vi "Main.vi"() -> ()   [LabVIEW 2021]
uses:
  Strict Type Controls/Command.ctl
  classes/Tushars Events Toolkit/Software/Modules/EventClient_ObjectReference.ctl
  Strict Type Controls/Settings Operation.ctl
  Strict Type Controls/Settings.ctl
  1f5d9b14-0bda-4edd-bf62-f35b82af222a.vi
  classes/Variable Manager/VariableManager_Bool.vi
  <vilib>/Utility/file.llb/Write To Spreadsheet File (string).vi
  classes/Variable Manager/VariableManager_Double.vi
  classes/Variable Manager/VariableManager_String.vi
panel:
  out "filterSetup?":bool
  out "Quit":bool
  out "error out":errorcluster
  in  "error in (no error)":errorcluster
  in  "abort":bool
  in  "start":bool
  out "gratSetup?":bool
  out "Status":string
  in  "Port Set":bool
  in  "Merlin":refnum<visa-resource-name>
  in  "Mono":refnum<visa-resource-name>
  out "statusFilter":bool
  in  "Start Filter Wheel":bool
  out "Agilent Current":dbl format="%#.4f A"
  out "Agilent Voltage":dbl format="%#.4f V"
  out "Test Status":bool
  out "statusMerlin":bool
  out "statusMC":bool
  out "statusPS":bool
  out "statusSM":bool
  in  "Start Merlin":bool
  in  "Start Monochromator":bool
  in  "Start Power Supply":bool
  in  "Start Source Meter":bool
  out "Merlin Voltage":dbl format="%#.7f mV"
  out "Measuring Wavelength":dbl format="%#.7f nm"
  out "Source Meter Voltage":dbl format="%#.7f mV"
  in  "tab":T1(tab)=enum."Script"
  in  "exportVT":bool
  out "VTGraph":cluster{dbl[], dbl[]}(graph)
  in  "Test Mode":enum16{"Time Mode", "dV/dt Mode"}(ring)
  in  "Log Interval":u32=50 min=100 step=1 format="%.0f mSec"
  in  "Test Time":dbl step=1.0 format="%<%H:%M:%S>t"
  out "Time Remaining":dbl format="%<%H:%M:%S>t"
  in  "Target dV/dt":dbl format="%#.9f mV"
  in  "Lock In time":dbl step=1.0 format="%<%H:%M:%S>t"
  out "dV/dt":dbl format="%#.11f mV"
  out "Locked Time":dbl step=1.0 format="%<%H:%M:%S>t"
  in  "Perform Test After":T1(ring)=enum."Voltage Vs Wavelength"
  out "Wave":bool
  out "Slit":bool
  out "Shutter":bool
  out "Filter":bool
  out "Gr.Den":bool
  in  "GratingNo":i32=1 min=1 max=3 step=1
  in  "Wavelen(nm)":i32
  in  "setWavelength":bool
  in  "SetGrating":bool
  in  "SetSlit":bool
  in  "Slit":i32=1 min=1 max=8 step=1
  out "Wavenumber":i32
  in  "Set Grating Density":bool
  in  "GratingDen":i32=1 min=1 max=2 step=1
  in  "Filter Set":bool
  in  "Filter Num":i32=1 min=1 max=5 step=1
  in  "Shutter":enum16{"Open", "Close"}(ring)
  in  "ShutterOp":bool
  in  "Filter Block":bool
  in  "Filter Disable":bool
  in  "Filter Enab":bool
  in  "Frequency":u32=15 min=8 max=1100 step=1
  in  "setMerlin":bool
  in  "#Filter Stages":enum16{"None", "1 Pole", "2 Pole"}(ring)
  in  "Phase":enum16{"1 Phase", "2 Phase"}(ring)
  in  "SyncMode":T2(ring)
  in  "Time Const":T3(ring)
  in  "setOffsets":bool
  in  "portD":bool
  in  "portA":bool
  in  "Settling Time (ms)":dbl=10000.0
  in  "To":i32=1000
  in  "Step":dbl=100.0
  in  "From":i32=200
  in  "exportSweep":bool
  out "sweep":cluster{dbl[], dbl[]}[](graph)
  in  "Slit":string(combo)
  in  "Sweep Results":i32(listbox)
  in  "Reset":bool
  out "Gr.no":bool
  out "Reset 2":bool
  in  "exportScriptWave":bool
  out "scriptSweep":cluster{dbl[], dbl[]}[](graph)
  in  "Command":T4
  in  "Parm 4":dbl format="%#.6f"
  in  "Parm 3":dbl format="%#.6f"
  in  "openScript":bool
  in  "exportScript":bool
  in  "update":bool
  out "scriptGraph":cluster{dbl[], dbl[]}(graph)
  in  "Parm 2":dbl format="%#.6f"
  in  "Parm 1":dbl format="%#.6f"
  in  "script":i32(listbox)
  in  "add":bool
  in  "remove":bool
  in  "exportScriptResults":bool
  in  "Script Avg Interval":u32=200 min=100 step=1 format="%.0f mSec"
  # "Status"
  # "Port Setting"
  # "NOTE:\n1. if this LED is OFF then GPIB is not connected...\n2. Close program before power off Instruments..."
  # "Test Type"
  # "Test Time"
  # "Voltage Results"
  # "Monochromator"
  # "Merlin"
  # "Merlin"
  # "Sweep"
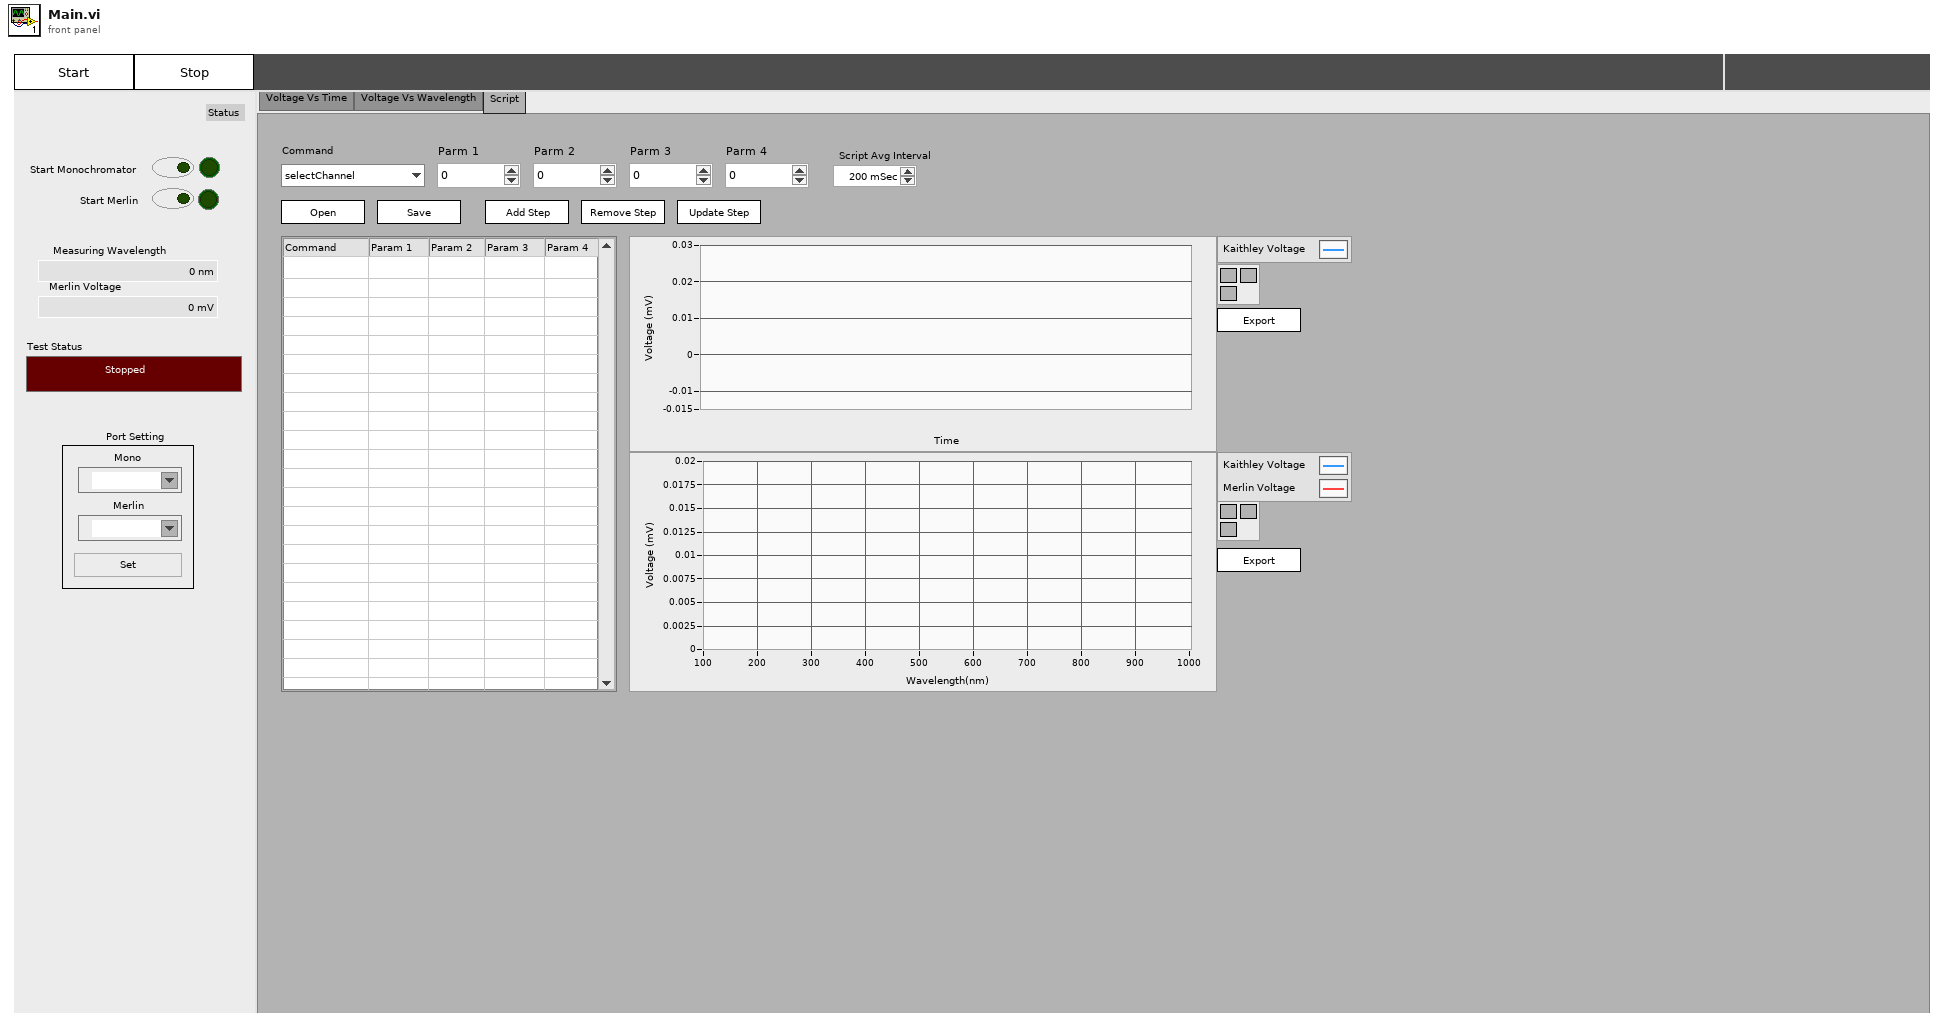
[diagram p1: front panel]
types:
  T1 = enum32{"Voltage Vs Time", "Voltage Vs Wavelength", "Script"}
  T2 = enum16{"Int Chop Off", "Int Chop On", "Ext Chop Off", "Ext Chop On"}
  T3 = enum16{".003s", ".010s", ".030s", ".100s", ".300s", "1.00s", "3.00s", "10.0s", "30.0s", "100s"}
  T4 = typedef "Command.ctl" = enum16{"selectChannel", "setDCVoltage", "setDCCurrent", "setVoltageSteps", "wait", "setWavelength", "setWavelengthSteps"}
  T5 = typedef "Settings Operation.ctl" = enum8{"Get Value", "Set Value", "Read File", "Write File", "Write Stored Value"}
  T6 = enum32{"invalid app kind", "Development System", "Run Time System", "Student Edition", "Embedded LabVIEW", "Evaluation", "Custom"}
  T7 = cluster{"startTime":u32, "lastUpdate":u32, "lastVoltage":dbl, "run?":bool, "From":i32, "time":dbl[], "MerlinVal":dbl[], "SMVolt":dbl[], "sweepType":enum16{"ASC", "DESC"}, "Wavlnth":dbl[], "Test Mode":enum16{"Time Mode", "dV/dt Mode"}, "tab":enum32{"Voltage Vs Time", "Voltage Vs Wavelength", "Script"}, "script":string[][], "dV/dt":dbl[], "graphUpdate":u32, "Filter Num":i32}
  T8 = typedef "EventClient_ObjectReference.ctl" = refnum<k1>
  T9 = typedef "Settings.ctl" = cluster{"Mono Cr":cluster{"Port":refnum<visa-resource-name>, "baud rate":u32, "data bits":u16, "parity":enum16{"None", "Odd", "Even", "Mark", "Space"}, "stop bits":u16, "flow control":u16, "timeout":u32}, "Merlin":cluster{"Port":refnum<visa-resource-name>, "baud rate":u32, "data bits":u16, "parity":enum16{"None", "Odd", "Even", "Mark", "Space"}, "stop bits":u16, "flow control":u16, "timeout":u32}}
  T10 = cluster{"#Stages":enum16{"None", "1 Pole", "2 Pole"}, "Phase":enum16{"1 Phase", "2 Phase"}, "SyncMode":enum16{"Int Chop Off", "Int Chop On", "Ext Chop Off", "Ext Chop On"}, "Time Const":enum16{".003s", ".010s", ".030s", ".100s", ".300s", "1.00s", "3.00s", "10.0s", "30.0s", "100s"}, "Frequency":u32}
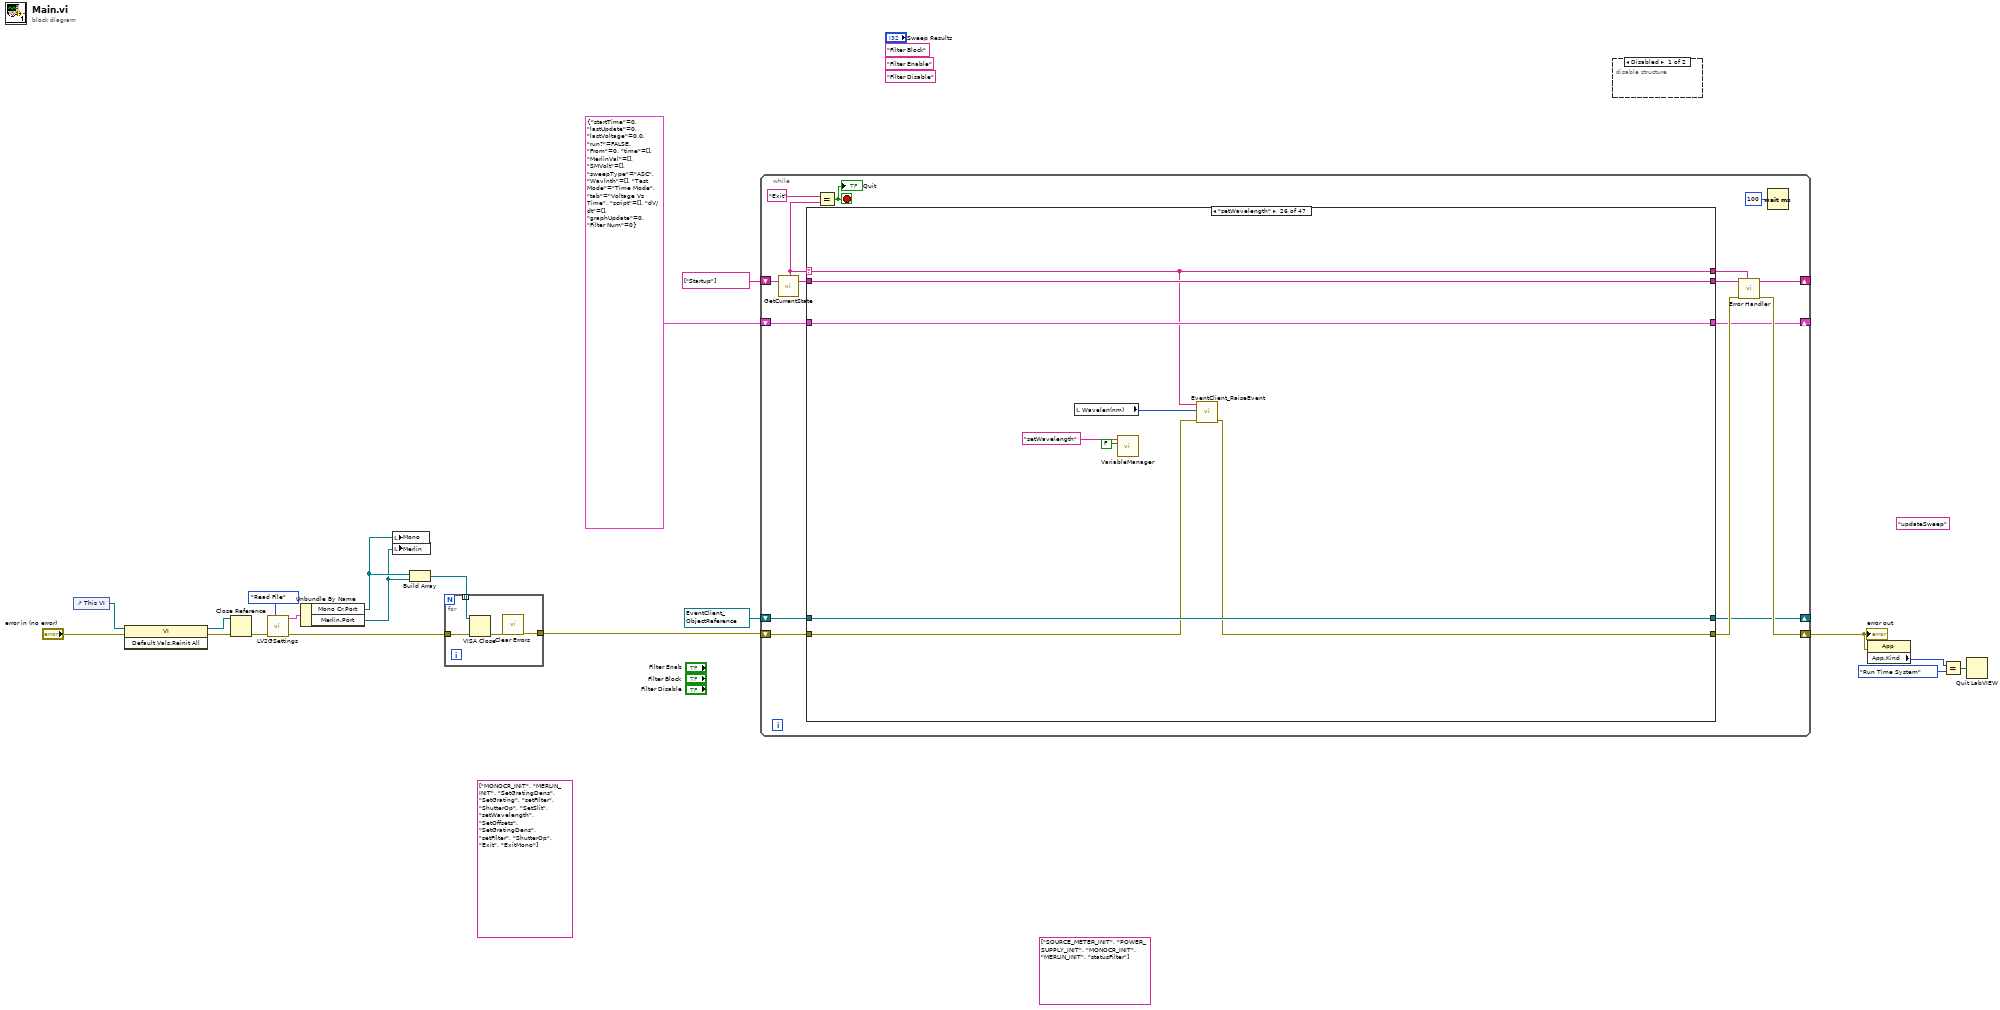
[diagram p0: block diagram]
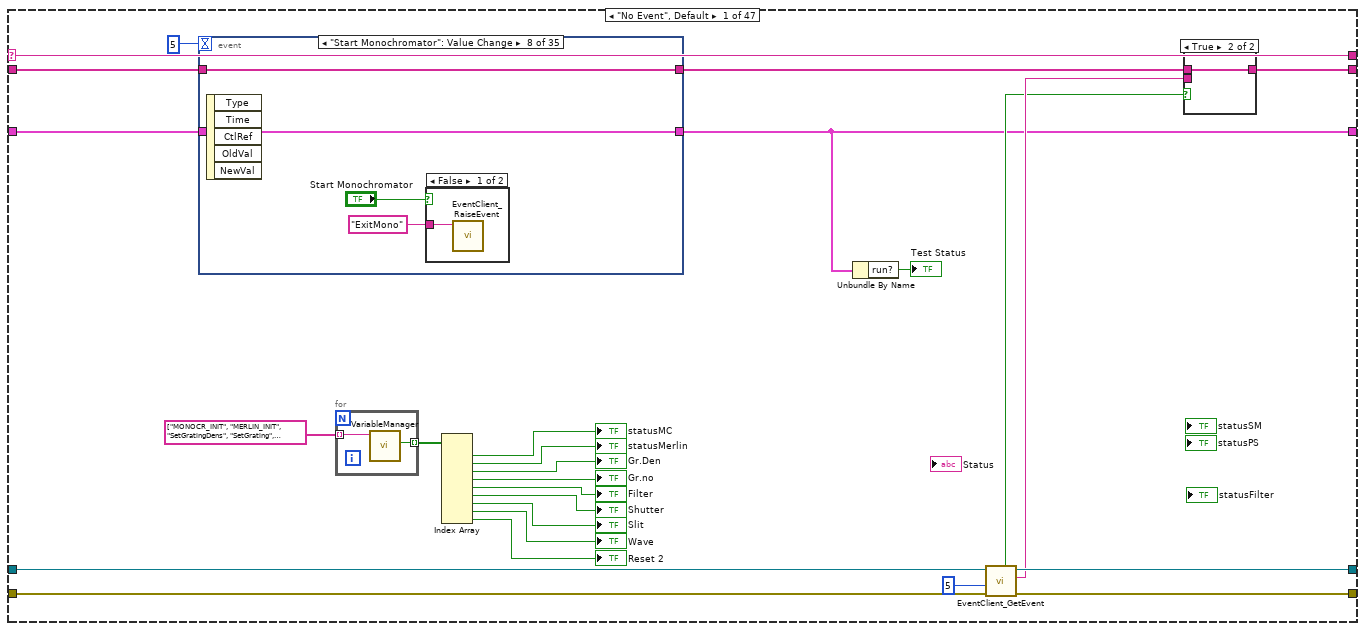
[diagram p3: hidden frame]
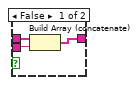
[diagram p4: hidden frame]
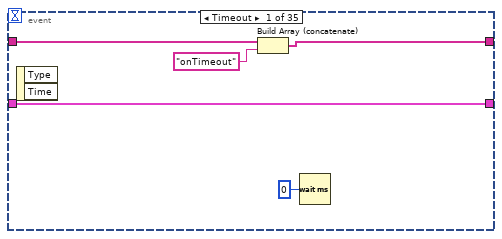
[diagram p5: hidden frame]
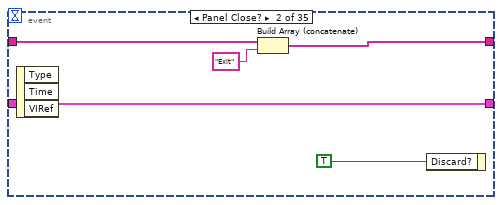
[diagram p6: hidden frame]
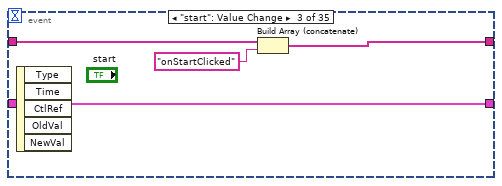
[diagram p7: hidden frame]
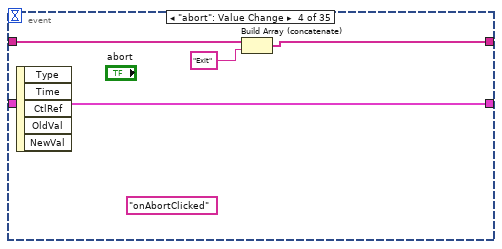
[diagram p8: hidden frame]
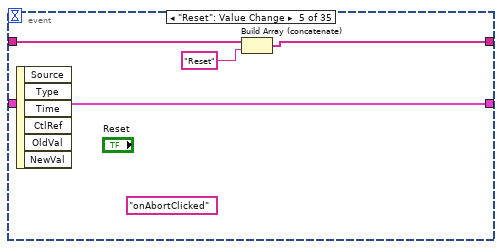
[diagram p9: hidden frame]
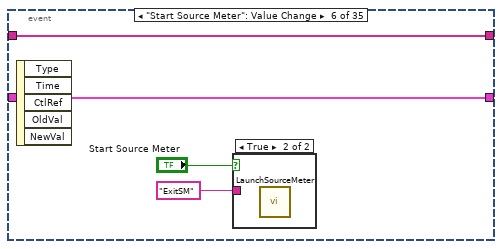
[diagram p10: hidden frame]
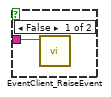
[diagram p11: hidden frame]
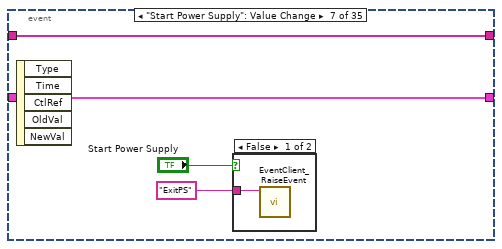
[diagram p12: hidden frame]
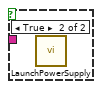
[diagram p13: hidden frame]
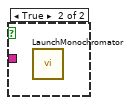
[diagram p14: hidden frame]
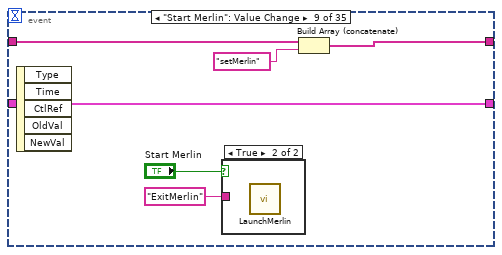
[diagram p15: hidden frame]
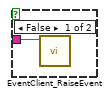
[diagram p16: hidden frame]
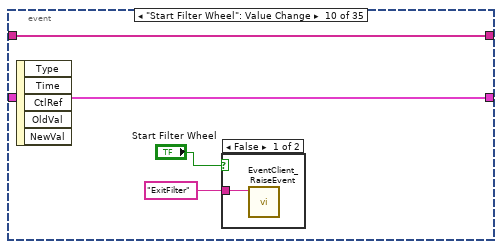
[diagram p17: hidden frame]
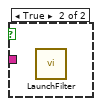
[diagram p18: hidden frame]
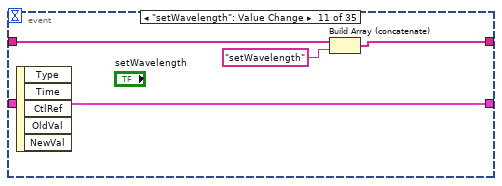
[diagram p19: hidden frame]
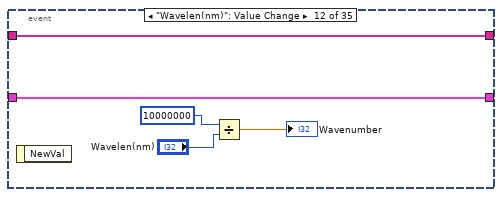
[diagram p20: hidden frame]
diagram:
  (unwired) "updateSweep" ("String")
  (unwired) string[] ["MONOCR_INIT", "MERLIN_INIT", "SetGratingDens", "SetGrating", "setFIlter", "ShutterOp", "SetSlit", "setWavelength", "SetOffsets", "SetGratingDens", "setFIlter", "ShutterOp", "Exit", "ExitMono"] ("Events")
  (unwired) string[] ["SOURCE_METER_INIT", "POWER_SUPPLY_INIT", "MONOCR_INIT", "MERLIN_INIT", "statusFilter"] ("State Array Out")
  (unwired) "Filter Block"
  (unwired) "Filter Disable"
  (unwired) "Filter Enable"
  w19 = T8 refnum items=["EventClient"] ("reference")
  n1 = control-ref of="This VI"() -> (w11:refnum<vi>)
  n2 = invoke class="VI" method="Default Vals.Reinit All"(reference=w11, error in="error in (no error)") -> (reference out=w9:refnum<vi>, error out=w10:errorcluster)  [unwired: 1 in, 1 out]
  n3 = Close Reference(reference=w9, error in (no error)=w10) -> (error out=w8:errorcluster)
  n4 = call "LV2GSettings.vi"("Operation"=Settings_Operation."Read File", "error in (no error)"=w8) -> ("error out"=w3:errorcluster, "Settings out"=w7:T9)  [unwired: 8 in]
  n5 = Unbundle By Name(w7) -> ("Mono Cr.Port"=w5:refnum<visa-resource-name>, "Merlin.Port"=w4:refnum<visa-resource-name>)
  n6 = local write "Mono"(w5) -> ()
  n7 = local write "Merlin"(w4) -> ()
  n8 = Build Array(w5, w4) -> (w2:refnum<visa-resource-name>[])
  n9 = for {
    tunnel: w3 -> [w22]
    tunnel: w2 -> [w23] mode=indexing
    tunnel: [w20] -> w1
    n10 = VISA Close(VISA resource name=w23, error in (no error)=w22) -> (error out=w21:errorcluster)
    n11 = call <vilib>:"Clear Errors.vi"("error in (no error)"=w21) -> ("error out"=w20:errorcluster)  [unwired: 5 in, 1 out]
  }
  n12 = while {
    shift-right: [w35] -> _
    shift-left: string[] ["Startup"] ("State Array Out") -> [w39]
    shift-right: [w31] -> w16
    shift-left: w1 -> [w32]
    shift-right: [w28] -> _
    shift-left: w19 -> [w27]
    shift-right: [w25] -> _
    shift-left: T7 {"startTime"=0, "lastUpdate"=0, "lastVoltage"=0.0, "run?"=FALSE, "From"=0, "time"=[], "MerlinVal"=[], "SMVolt"=[], "sweepType"=enum."ASC", "Wavlnth"=[], "Test Mode"=enum."Time Mode", "tab"=enum."Voltage Vs Time", "script"=[], "dV/dt"=[], "graphUpdate"=0, "Filter Num"=0} -> [w26]
    stop <- w36 stop-if-true
    n13 = call "GetCurrentState.vi"("State Array In"=w39) -> ("Current State"=w29:string, "State Array Out"=w38:string[])  [unwired: 17 in]
    n14 = case shown="\"setWavelength\"" w29 {
      selector: w29 -> [w65 w246 w258 w268 w273 w278 w283 w288 w306 w322 w345 w372 w390 w401 w422 w439 w447 w477 w495 w506 w518 w526 w532 w541 w552 w561 w571 w579 w588 w604 w617 w623 w633 w662 w673 w678 w699 w754 w774 w804 w836 w864 w922 w984 w1019 w1048 w1064]
      tunnel: w38 -> [w64 w245 w264 w269 w274 w279 w284 w289 w307 w323 w346 w373 w391 w402 w423 w440 w448 w450 w496 w507 w519 w527 w536 w545 w556 w565 w574 w583 w592 w608 w619 w624 w634 w663 w674 w679 w690 w737 w758 w796 w828 w855 w901 w985 w1020 w1047 w1051]
      tunnel: [w55 w244 w264 w269 w274 w279 w284 w289 w307 w323 w346 w373 w391 w402 w423 w440 w448 w449 w496 w507 w519 w527 w536 w545 w556 w565 w574 w583 w592 w608 w619 w624 w634 w663 w674 w679 w691 w736 w757 w795 w830 w854 w900 w973 w1020 w1047 w1051] -> w34
      tunnel: [w60 w238 w259 w267 w272 w277 w282 w287 w305 w321 w344 w371 w389 w400 w421 w438 w446 w476 w494 w505 w512 w520 w533 w542 w553 w559 w568 w577 w587 w605 w614 w622 w629 w658 w669 w677 w698 w753 w773 w803 w835 w862 w902 w980 w1018 w1046 errorcluster {"status"=FALSE, "code"=0, "source"=""} ("error in (no error)")] -> w30
      tunnel: [w65 w246 w258 w268 w273 w278 w283 w288 w306 w322 w345 w372 w390 w401 w422 w439 w447 w477 w495 w506 w518 w526 w532 w541 w552 w561 w571 w579 w588 w604 w617 w623 w633 w662 w673 w678 w699 w754 w774 w804 w836 w864 w922 w984 w1019 w1048 w1064] -> w33
      tunnel: w32 -> [w61 w226 w262 w267 w272 w277 w282 w287 w305 w321 w344 w371 w389 w400 w421 w438 w446 w476 w494 w505 w513 w521 w534 w543 w554 w560 w570 w580 w589 w606 w615 w622 w631 w660 w671 w677 w698 w753 w773 w803 w835 w862 w903 w981 w1018 w1046 w1052]
      tunnel: [w59 w236 w261 w266 w271 w276 w281 w286 w304 w320 w343 w370 w388 w399 w420 w437 w445 w475 w493 w504 w517 w525 w535 w544 w555 w564 w573 w582 w591 w607 w618 w621 w627 w656 w667 w676 w697 w752 w772 w802 w834 w863 w921 w983 w1017 w1045 w1050] -> w28
      tunnel: w27 -> [w62 _ w263 w266 w271 w276 w281 w286 w304 w320 w343 w370 w388 w399 w420 w437 w445 w475 w493 w504 w517 w525 w535 w544 w555 w564 w573 w582 w591 w607 w618 w621 w632 w661 w672 w676 w697 w752 w772 w802 w834 w863 w921 w983 w1017 w1045 w1050]
      tunnel: w26 -> [w53 w234 w257 w265 w270 w275 w280 w285 w303 w319 w342 w369 w387 w398 w419 w436 w444 w474 w492 w503 w516 w524 w530 w540 w551 w563 w572 w581 w590 w597 w616 w620 w625 w655 w666 w675 w696 w742 w771 w800 w833 w857 w920 w971 w1010 w1044 w1049]
      tunnel: [w52 w234 w257 w265 w270 w275 w280 w285 w303 w319 w342 w369 w387 w398 w419 w436 w444 w473 w491 w503 w516 w524 w530 w540 w551 w563 w572 w581 w590 w597 w616 w620 w625 w655 w666 w675 w696 w741 w768 w798 w833 w856 w919 w982 w1009 w1044 w1049] -> w25
      frame "No Event", Default {
        n15 = event shown="[7] \"Start Monochromator\": Value Change" {
          selector: _ -> [_ _ _ _ _ _ _ _ _ _ _ _ _ _ _ _ _ _ _ _ _ _ _ _ _ _ _ _ _ _ _ _ _ _ _]
          dyn-events: _ -> [_ _ _ _ _ _ _ _ _ _ _ _ _ _ _ _ _ _ _ _ _ _ _ _ _ _ _ _ _ _ _ _ _ _ _]
          timeout: 5 -> [_ _ _ _ _ _ _ _ _ _ _ _ _ _ _ _ _ _ _ _ _ _ _ _ _ _ _ _ _ _ _ _ _ _ _]
          tunnel: [w74 w79 w84 w88 w92 w97 w102 w107 w110 w119 w123 w129 w132 w136 w140 w144 w147 w151 w155 w159 w163 w167 w171 w175 w179 w183 w187 w191 w195 w199 w203 w207 w211 w215 w219] -> w56
          tunnel: w64 -> [w76 w81 w85 w89 w93 w97 w102 w107 w114 w119 w124 w129 w133 w137 w141 w145 w148 w152 w156 w159 w164 w168 w172 w176 w180 w184 w188 w192 w196 w200 w204 w208 w212 w216 w220]
          tunnel: w53 -> [w75 w77 w82 w87 w91 w96 w101 w106 w113 w118 w121 w128 w130 w134 w138 w142 w149 w153 w157 w160 w161 w165 w169 w173 w177 w181 w185 w189 w193 w197 w201 w205 w209 w213 w217]
          tunnel: [w75 w77 w82 w87 w91 w96 w101 w106 w113 w118 w121 w128 w130 w134 w138 w142 w149 w153 w157 w160 w161 w165 w169 w173 w177 w181 w185 w189 w193 w197 w201 w205 w209 w213 w217] -> w52
          event Timeout {
            n16 = event-data() -> ()  [unwired: 1 in, 2 out]
            n17 = Build Array (concatenate)(w76, "onTimeout" ("x")) -> (w74:string[])
            n18 = Wait (ms)(milliseconds to wait=u32 0) -> ()  [unwired: 1 out]
          }
          event Panel Close? {
            n19 = event-data() -> ()  [unwired: 1 in, 3 out]
            n20 = Build Array (concatenate)(w81, "Exit" ("x")) -> (w79:string[])
            n21 = event-data("Discard?"=TRUE) -> ()  [unwired: 1 in, 1 out]
          }
          event "start": Value Change {
            n22 = event-data() -> ()  [unwired: 1 in, 5 out]
            n23 = Build Array (concatenate)(w85, "onStartClicked" ("x")) -> (w84:string[])
          }
          event "abort": Value Change {
            (unwired) "onAbortClicked" ("x")
            n24 = event-data() -> ()  [unwired: 1 in, 5 out]
            n25 = Build Array (concatenate)(w89, "Exit" ("x")) -> (w88:string[])
          }
          event "Reset": Value Change {
            (unwired) "onAbortClicked" ("x")
            n26 = event-data() -> ()  [unwired: 1 in, 6 out]
            n27 = Build Array (concatenate)(w93, "Reset" ("x")) -> (w92:string[])
          }
          event "Start Source Meter": Value Change {
            n28 = event-data() -> ()  [unwired: 1 in, 5 out]
            n29 = case shown="True" "Start Source Meter" {
              tunnel: "ExitSM" -> [w98 _]
              frame False {
                n30 = call "EventClient_RaiseEvent.vi"("Event"=w98) -> ()  [unwired: 10 in, 1 out]
              }
              frame True {
                n31 = call "LaunchSourceMeter.vi"() -> ()  [unwired: 11 in, 1 out]
              }
            }
          }
          event "Start Power Supply": Value Change {
            n32 = event-data() -> ()  [unwired: 1 in, 5 out]
            n33 = case shown="False" "Start Power Supply" {
              tunnel: "ExitPS" -> [w103 _]
              frame False {
                n34 = call "EventClient_RaiseEvent.vi"("Event"=w103) -> ()  [unwired: 10 in, 1 out]
              }
              frame True {
                n35 = call "LaunchPowerSupply.vi"() -> ()  [unwired: 11 in, 1 out]
              }
            }
          }
          event "Start Monochromator": Value Change {
            n36 = event-data() -> ()  [unwired: 1 in, 5 out]
            n37 = case shown="False" "Start Monochromator" {
              tunnel: "ExitMono" -> [w108 _]
              frame False {
                n38 = call "EventClient_RaiseEvent.vi"("Event"=w108) -> ()  [unwired: 10 in, 1 out]
              }
              frame True {
                n39 = call "LaunchMonochromator.vi"() -> ()  [unwired: 11 in, 1 out]
              }
            }
          }
          event "Start Merlin": Value Change {
            n40 = event-data() -> ()  [unwired: 1 in, 5 out]
            n41 = case shown="True" "Start Merlin" {
              tunnel: "ExitMerlin" -> [w115 _]
              frame False {
                n42 = call "EventClient_RaiseEvent.vi"("Event"=w115) -> ()  [unwired: 10 in, 1 out]
              }
              frame True {
                n43 = call "LaunchMerlin.vi"() -> ()  [unwired: 11 in, 1 out]
              }
            }
            n44 = Build Array (concatenate)(w114, "setMerlin") -> (w110:string[])
          }
          event "Start Filter Wheel": Value Change {
            n45 = event-data() -> ()  [unwired: 1 in, 5 out]
            n46 = case shown="False" "Start Filter Wheel" {
              tunnel: "ExitFilter" -> [w120 _]
              frame False {
                n47 = call "EventClient_RaiseEvent.vi"("Event"=w120) -> ()  [unwired: 10 in, 1 out]
              }
              frame True {
                n48 = call "LaunchFilter.vi"() -> ()  [unwired: 11 in, 1 out]
              }
            }
          }
          event "setWavelength": Value Change {
            n49 = event-data() -> ()  [unwired: 1 in, 5 out]
            n50 = Build Array (concatenate)(w124, "setWavelength" ("x")) -> (w123:string[])
          }
          event "Wavelen(nm)": Value Change {
            n51 = event-data() -> ()  [unwired: 1 in, 1 out]
            n52 = Divide(x=10000000 ("y"), y="Wavelen(nm)") -> (x/y=→"Wavenumber":dbl)
          }
          event "SetGrating": Value Change {
            n53 = event-data() -> ()  [unwired: 1 in, 5 out]
            n54 = Build Array (concatenate)(w133, "SetGrating" ("x")) -> (w132:string[])
          }
          event "Set Grating Density": Value Change {
            n55 = event-data() -> ()  [unwired: 1 in, 5 out]
            n56 = Build Array (concatenate)(w137, "SetGratingDens" ("x")) -> (w136:string[])
          }
          event "Filter Set": Value Change {
            n57 = event-data() -> ()  [unwired: 1 in, 5 out]
            n58 = Build Array (concatenate)(w141, "setFIlter" ("x")) -> (w140:string[])
          }
          event "ShutterOp": Value Change {
            n59 = event-data() -> ()  [unwired: 1 in, 5 out]
            n60 = Build Array (concatenate)(w145, "ShutterOp" ("x")) -> (w144:string[])
          }
          event "Filter Enab": Value Change {
            n61 = event-data() -> ()  [unwired: 1 in, 6 out]
            n62 = Build Array (concatenate)(w148, "Filter Enable") -> (w147:string[])
          }
          event "Filter Disable": Value Change {
            n63 = event-data() -> ()  [unwired: 1 in, 6 out]
            n64 = Build Array (concatenate)(w152, "Filter Disable") -> (w151:string[])
          }
          event "Filter Block": Value Change {
            n65 = event-data() -> ()  [unwired: 1 in, 6 out]
            n66 = Build Array (concatenate)(w156, "Filter Block") -> (w155:string[])
          }
          event "setOffsets": Value Change {
            n67 = event-data() -> ()  [unwired: 1 in, 5 out]
            n68 = call "EventClient_RaiseEvent.vi"("Event"="SetOffsets") -> ()  [unwired: 10 in, 1 out]
          }
          event "SetSlit": Value Change {
            n69 = event-data() -> ()  [unwired: 1 in, 5 out]
            n70 = Build Array (concatenate)(w164, "SetSlit" ("x")) -> (w163:string[])
          }
          event "setMerlin", "Frequency": Value Change {
            n71 = event-data() -> ()  [unwired: 1 in, 2 out]
            n72 = Build Array (concatenate)(w168, "setMerlin" ("x")) -> (w167:string[])
          }
          event "exportSweep": Value Change {
            n73 = event-data() -> ()  [unwired: 1 in, 5 out]
            n74 = Build Array (concatenate)(w172, "exportSweep" ("x")) -> (w171:string[])
          }
          event "exportVT": Value Change {
            n75 = event-data() -> ()  [unwired: 1 in, 5 out]
            n76 = Build Array (concatenate)(w176, "exportVT" ("x")) -> (w175:string[])
          }
          event "portA": Value Change {
            n77 = event-data() -> ()  [unwired: 1 in, 5 out]
            n78 = Build Array (concatenate)(w180, "portA" ("x")) -> (w179:string[])
          }
          event "portD": Value Change {
            n79 = event-data() -> ()  [unwired: 1 in, 5 out]
            n80 = Build Array (concatenate)(w184, "portD" ("x")) -> (w183:string[])
          }
          event "add": Value Change {
            n81 = event-data() -> ()  [unwired: 1 in, 5 out]
            n82 = Build Array (concatenate)(w188, "addStep" ("x")) -> (w187:string[])
          }
          event "remove": Value Change {
            n83 = event-data() -> ()  [unwired: 1 in, 5 out]
            n84 = Build Array (concatenate)(w192, "removeStep" ("x")) -> (w191:string[])
          }
          event "update": Value Change {
            n85 = event-data() -> ()  [unwired: 1 in, 5 out]
            n86 = Build Array (concatenate)(w196, "updateStep" ("x")) -> (w195:string[])
          }
          event "exportScript": Value Change {
            n87 = event-data() -> ()  [unwired: 1 in, 5 out]
            n88 = Build Array (concatenate)(w200, "exportScript" ("x")) -> (w199:string[])
          }
          event "exportScriptResults": Value Change {
            n89 = event-data() -> ()  [unwired: 1 in, 5 out]
            n90 = Build Array (concatenate)(w204, "exportScriptResults" ("x")) -> (w203:string[])
          }
          event "exportScriptWave": Value Change {
            n91 = event-data() -> ()  [unwired: 1 in, 5 out]
            n92 = Build Array (concatenate)(w208, "exportScriptWave" ("x")) -> (w207:string[])
          }
          event "openScript": Value Change {
            n93 = event-data() -> ()  [unwired: 1 in, 5 out]
            n94 = Build Array (concatenate)(w212, "openScript" ("x")) -> (w211:string[])
          }
          event "script": Value Change {
            n95 = event-data() -> ()  [unwired: 1 in, 5 out]
            n96 = Build Array (concatenate)(w216, "onScriptRowSelected" ("x")) -> (w215:string[])
          }
          event "Port Set": Value Change {
            n97 = event-data() -> ()  [unwired: 1 in, 6 out]
            n98 = Build Array (concatenate)(w220, "Port set" ("x")) -> (w219:string[])
          }
        }
        n99 = for {
          tunnel: string[] ["MONOCR_INIT", "MERLIN_INIT", "SetGratingDens", "SetGrating", "setFIlter", "ShutterOp", "SetSlit", "setWavelength", "Exit", "ExitMono", "Reset"] ("Events") -> [w67] mode=indexing
          tunnel: [w66] -> w50 mode=indexing
          n100 = call-poly "VariableManager.vi"("Tag"=w67) -> ("Value out"=w66:bool)  [unwired: 7 in, 3 out]
        }
        n101 = Index Array(array=w50) -> (element #1=→"statusMC":bool, element #2=→"statusMerlin":bool, element #3=→"Gr.Den":bool, element #4=→"Gr.no":bool, element #5=→"Filter":bool, element #6=→"Shutter":bool, element #7=→"Slit":bool, element #8=→"Wave":bool, element #9=→"Reset 2":bool)  [unwired: 9 in]
        n102 = Unbundle By Name(w52) -> ("run?"=→"Test Status":bool)
        n103 = call "EventClient_GetEvent.vi"("error in (no error)"=w61, "timeout in ms (-1)"=5, "reference"=w62) -> ("error out"=w60:errorcluster, "Name"=w58:string, "reference out"=w59:T8, "timed out?"=w57:bool)  [unwired: 4 in, 1 out]
        n104 = case shown="True" w57 {
          tunnel: w56 -> [w70 w71]
          tunnel: w58 -> [w69 _]
          tunnel: [w68 w71] -> w55
          frame False {
            n105 = Build Array (concatenate)(w70, w69) -> (w68:string[])
          }
          frame True {
          }
        }
      }
      frame "Startup" {
        w224 = cluster{dbl[], dbl[]}[] [] ("sweep")
        w225 = cluster{dbl[], dbl[]} {[], []} ("VTGraph")
        w229 = string[] ["Command", "Param 1", "Param 2", "Param 3", "Param 4"]  # script
        w222 = FALSE ("Start Source Meter")
        w223 = u32 200 ("Log Interval")
        # "If Multiple instnances of this VI are possible \nthen make sure that client created in each instance gets a different Name"
        n106 = local write "Script Avg Interval"(w223) -> ()
        n107 = local write "Log Interval"(w223) -> ()
        n108 = local write "Test Time"(90.0 ("Locked Time")) -> ()
        n109 = local write "Target dV/dt"(1.0 ("Target dV/dt")) -> ()
        n110 = local write "Lock In time"(30.0 ("Lock In time")) -> ()
        n111 = local write "VTGraph"(w225) -> ()
        n112 = local write "scriptGraph"(w225) -> ()
        n113 = local write "scriptSweep"(w224) -> ()
        n114 = local write "sweep"(w224) -> ()
        n115 = local write "tab"(T1."Voltage Vs Wavelength" ("tab")) -> ()
        n116 = disable-structure shown="Enabled" {
          disable-tunnel: [w255 w256] -> w230
          disable-tunnel: w226 -> [w254 w256]
          frame Disabled {
            n117 = call "LaunchPowerSupply.vi"("error in (no error)"=w254) -> ("error out"=w253:errorcluster)  [unwired: 10 in]
            n118 = call "LaunchSourceMeter.vi"("error in (no error)"=w253) -> ("error out"=w252:errorcluster)  [unwired: 10 in]
            n119 = call "LaunchMerlin.vi"("error in (no error)"=w252) -> ("error out"=w251:errorcluster)  [unwired: 10 in]
            n120 = call "LaunchMonochromator.vi"("error in (no error)"=w251) -> ("error out"=w255:errorcluster)  [unwired: 10 in]
          }
          frame Enabled {
          }
        }
        n121 = for {
          tunnel: string[] ["MONOCR_INIT", "MERLIN_INIT", "SetGratingDens", "SetGrating", "setFIlter", "ShutterOp", "SetSlit", "setWavelength", "SetOffsets", "SetGratingDens", "setFIlter", "ShutterOp", "Exit", "ExitMono"] ("Events") -> [w250] mode=indexing
          tunnel: [w249] -> _ mode=indexing
          n122 = call-poly "VariableManager.vi"("Operation"=enum16{"Get Tag", "Set Tag"}."Set Tag", "Value"=FALSE, "Tag"=w250) -> ("Value out"=w249:bool)  [unwired: 5 in, 3 out]
        }
        n123 = Call Chain() -> (call chain=w242:string[])
        n124 = Index Array(array=w242, index=0) -> (element=w240:string)
        n125 = call "EventClient_Create.vi"("error in (no error)"=w230, "Instance Name"=w240) -> ("error out"=w239:errorcluster, "reference"=w237:T8)  [unwired: 8 in]
        n126 = Build Array (concatenate)(w245, string[] [] ("State Array Out")) -> (w244:string[])
        n127 = call "EventClient_SubscribeEvents.vi"("error in (no error)"=w239, "Events"=string[] ["currGrating", "updateScriptSweep"], "reference"=w237) -> ("error out"=w238:errorcluster, "reference out"=w236:T8)  [unwired: 7 in]
        n128 = local write "Start Source Meter"(w222) -> ()
        n129 = local write "Start Power Supply"(w222) -> ()
        n130 = local write "Start Monochromator"(w222) -> ()
        n131 = local write "Start Merlin"(w222) -> ()
        n132 = local write "statusMC"(w222) -> ()
        n133 = property on="script" class="MCListbox (strict)"("ColHdrString"=w229, "ItemNames"=string[][] [] ("Item Names")) -> ()  [unwired: 2 in, 2 out]
      }
      frame "Exit" {
        w261 = T8 refnum items=["EventClient"] ("reference out")
        n134 = call "EventClient_Destroy.vi"("error in (no error)"=w262, "reference"=w263) -> ("error out"=w260:errorcluster)  [unwired: 9 in]
        n135 = call "EventClient_RaiseEvent.vi"("error in (no error)"=w260, "Event"=w258) -> ("error out"=w259:errorcluster)  [unwired: 9 in]
      }
      frame "---------------Filter operation---------------" {
        # "This State will never Execute\nIt is added just for improving code readability please do not remove this case"
      }
      frame "Filter Enable" {
      }
      frame "Filter Disable" {
      }
      frame "Filter Block" {
      }
      frame "---------------Below are UI Events---------------" {
        # "This State will never Execute\nIt is added just for improving code readability please do not remove this case"
      }
      frame "onScriptRowSelected" {
        w295 = 0 ("index")
        n136 = property on="script" class="MCListbox (strict)"() -> ("ItemNames"=w302:string[][], "Value"=w301:i32)  [unwired: 2 in, 2 out]
        n137 = Index Array(array=w302, index (row)=w301) -> (element=w299:string[])  [unwired: 1 in]
        n138 = Delete From Array(array=w299, index=w295) -> (deleted portion=w298:string, array with subset deleted=w300:string[])  [unwired: 1 in]
        n139 = Scan From String(input string=w298, default 1=Command."selectChannel" ("Command")) -> (output 1=w294:T4)  [unwired: 3 in, 3 out]
        n140 = Fract/Exp String To Number(string=w300) -> (number=w296:dbl[])  [unwired: 3 in, 1 out]
        n141 = Index Array(array=w296, index #1=w295) -> (element #1=w293:dbl, element #2=w292:dbl, element #3=w291:dbl, element #4=w290:dbl)  [unwired: 3 in]
        n142 = local write "Parm 1"(w293) -> ()
        n143 = local write "Parm 2"(w292) -> ()
        n144 = local write "Parm 3"(w291) -> ()
        n145 = local write "Parm 4"(w290) -> ()
        n146 = local write "Command"(w294) -> ()
      }
      frame "exportVT" {
        n147 = local read "VTGraph"() -> (w313:cluster{dbl[], dbl[]})
        n148 = Unbundle(w313) -> (w317:dbl[], w314:dbl[])
        n149 = for {
          tunnel: w317 -> [w328] mode=indexing
          tunnel: "%<%H:%M:%S>t" ("format string") -> [w330]
          tunnel: [w329] -> w316 mode=indexing
          n150 = Format Into String(format string=w330, w328) -> (resulting string=w329:string)  [unwired: 2 in, 1 out]
        }
        n151 = Number To Fractional String(number=w314) -> (F-format string=w315:string[])  [unwired: 3 in]
        n152 = Build Array(w316, w315) -> (w312:string[][])
        n153 = call "File Dialog2"("pattern (all files)"="*.csv") -> ("selected path"=w311:path, "error out"=w310:errorcluster)  [unwired: 11 in, 2 out]
        n154 = Transpose 2D Array(2D array=w312) -> (transposed array=w308:string[][])
        n155 = case shown="Error" w310 {
          selector: w310 -> [_ w327]
          tunnel: w311 -> [w325 _]
          tunnel: w308 -> [w324 _]
          frame No Error {
            n156 = call-poly <vilib>:"Write To Spreadsheet File.vi"("delimiter (\\t)"="," ("delimiter (\\t)"), "2D data"=w324, "file path (dialog if empty)"=w325) -> ()  [unwired: 5 in, 1 out]
          }
          frame Error {
            n157 = call <vilib>:"Clear Errors.vi"("error in (no error)"=w327) -> ()  [unwired: 5 in, 2 out]
          }
        }
      }
      frame "exportScriptResults" {
        n158 = local read "scriptGraph"() -> (w337:cluster{dbl[], dbl[]})
        n159 = Unbundle(w337) -> (w340:dbl[], w336:dbl[])
        n160 = for {
          tunnel: w340 -> [w351] mode=indexing
          tunnel: "%<%H:%M:%S>t" ("format string") -> [w353]
          tunnel: [w352] -> w339 mode=indexing
          n161 = Format Into String(format string=w353, w351) -> (resulting string=w352:string)  [unwired: 2 in, 1 out]
        }
        n162 = Number To Fractional String(number=w336) -> (F-format string=w338:string[])  [unwired: 3 in]
        n163 = Build Array(w339, w338) -> (w335:string[][])
        n164 = Transpose 2D Array(2D array=w335) -> (transposed array=w331:string[][])
        n165 = call "File Dialog3"("pattern (all files)"="*.csv") -> ("selected path"=w334:path, "error out"=w333:errorcluster)  [unwired: 11 in, 2 out]
        n166 = case shown="No Error" w333 {
          selector: w333 -> [_ w350]
          tunnel: w334 -> [w348 _]
          tunnel: w331 -> [w347 _]
          frame No Error {
            n167 = call-poly <vilib>:"Write To Spreadsheet File.vi"("delimiter (\\t)"="," ("delimiter (\\t)"), "2D data"=w347, "file path (dialog if empty)"=w348) -> ()  [unwired: 5 in, 1 out]
          }
          frame Error {
            n168 = call <vilib>:"Clear Errors.vi"("error in (no error)"=w350) -> ()  [unwired: 5 in, 2 out]
          }
        }
      }
      frame "exportScriptWave" {
        (unwired) "%<%H:%M:%S>t" ("format string")
        n169 = local read "scriptSweep"() -> (w366:cluster{dbl[], dbl[]}[])
        n170 = Index Array(array=w366, index #1=0 ("index")) -> (element #1=w365:cluster{dbl[], dbl[]}, element #2=w363:cluster{dbl[], dbl[]})  [unwired: 1 in]
        n171 = Unbundle(w365) -> (w354:dbl[], w356:dbl[])
        n172 = Unbundle(w363) -> (w362:dbl[])  [unwired: 1 out]
        n173 = Number To Fractional String(number=w354) -> (F-format string=w355:string[])  [unwired: 3 in]
        n174 = Number To Fractional String(number=w356) -> (F-format string=w368:string[])  [unwired: 3 in]
        n175 = Number To Fractional String(number=w362) -> (F-format string=w361:string[])  [unwired: 3 in]
        n176 = Build Array(w355, w368, w361) -> (w367:string[][])
        n177 = Transpose 2D Array(2D array=w367) -> (transposed array=w357:string[][])
        n178 = call "File Dialog4"("pattern (all files)"="*.csv") -> ("selected path"=w360:path, "error out"=w359:errorcluster)  [unwired: 11 in, 2 out]
        n179 = case shown="No Error" w359 {
          selector: w359 -> [_ w377]
          tunnel: w360 -> [w375 _]
          tunnel: w357 -> [w374 _]
          frame No Error {
            n180 = call-poly <vilib>:"Write To Spreadsheet File.vi"("delimiter (\\t)"="," ("delimiter (\\t)"), "2D data"=w374, "file path (dialog if empty)"=w375) -> ()  [unwired: 5 in, 1 out]
          }
          frame Error {
            n181 = call <vilib>:"Clear Errors.vi"("error in (no error)"=w377) -> ()  [unwired: 5 in, 2 out]
          }
        }
      }
      frame "openScript" {
        w382 = string[][] []  # script
        n182 = Read from Text File() -> (text=w385:string, error out=w378:errorcluster)  [unwired: 4 in, 2 out]
        n183 = call <vilib>:"Clear Errors.vi"("error in (no error)"=w378) -> ()  [unwired: 5 in, 2 out]
        n184 = Spreadsheet String To Array(delimiter (Tab)=",", format string="%s", spreadsheet string=w385, array type (2D Dbl)=w382) -> (array=w381:string[][])
        n185 = Delete From Array(array=w381, index (row)=0) -> (deleted portion=w379:string[], array with subset deleted=w380:string[][])  [unwired: 2 in]
        n186 = property on="script" class="MCListbox (strict)"("ItemNames"=w380, "ColHdrString"=w379) -> ()  [unwired: 2 in, 2 out]
      }
      frame "exportScript" {
        n187 = property on="script" class="MCListbox (strict)"() -> ("ColHdrString"=w397:string[], "ItemNames"=w396:string[][])  [unwired: 2 in, 2 out]
        n188 = Build Array (concatenate)(w397, w396) -> (w392:string[][])
        n189 = call "File Dialog5"("pattern (all files)"="*.csv") -> ("selected path"=w395:path, "error out"=w394:errorcluster)  [unwired: 11 in, 2 out]
        n190 = case shown="No Error" w394 {
          selector: w394 -> [_ w406]
          tunnel: w395 -> [w404 _]
          tunnel: w392 -> [w403 _]
          frame No Error {
            n191 = call-poly <vilib>:"Write To Spreadsheet File.vi"("delimiter (\\t)"="," ("delimiter (\\t)"), "2D data"=w403, "file path (dialog if empty)"=w404) -> ()  [unwired: 5 in, 1 out]
          }
          frame Error {
            n192 = call <vilib>:"Clear Errors.vi"("error in (no error)"=w406) -> ()  [unwired: 5 in, 2 out]
          }
        }
      }
      frame "addStep" {
        n193 = Build Array("Parm 1", "Parm 2", "Parm 3", "Parm 4") -> (w413:dbl[])
        n194 = Format Into String("Command") -> (resulting string=w412:string)  [unwired: 3 in, 1 out]
        n195 = Number To Fractional String(number=w413, width (-)=i16 3 ("precision (6)")) -> (F-format string=w411:string[])  [unwired: 2 in]
        n196 = property on="script" class="MCListbox (strict)"() -> ("ItemNames"=w416:string[][])  [unwired: 2 in, 2 out]
        n197 = Build Array (concatenate)(w412, w411) -> (w410:string[])
        n198 = Build Array (concatenate)(w416, w410) -> (w415:string[][])
        n199 = property on="script" class="MCListbox (strict)"("ItemNames"=w415) -> ()  [unwired: 2 in, 2 out]
      }
      frame "updateStep" {
        n200 = local read "Command"() -> (w429:T4)
        n201 = local read "Parm 1"() -> (w428:dbl)
        n202 = local read "Parm 2"() -> (w427:dbl)
        n203 = local read "Parm 3"() -> (w425:dbl)
        n204 = local read "Parm 4"() -> (w424:dbl)
        n205 = Format Into String(w429) -> (resulting string=w431:string)  [unwired: 3 in, 1 out]
        n206 = Build Array(w428, w427, w425, w424) -> (w432:dbl[])
        n207 = property on="script" class="MCListbox (strict)"() -> ("ItemNames"=w435:string[][], "Value"=w433:i32)  [unwired: 2 in, 2 out]
        n208 = Number To Fractional String(number=w432) -> (F-format string=w430:string[])  [unwired: 3 in]
        n209 = Build Array (concatenate)(w431, w430) -> (w426:string[])
        n210 = Replace Array Subset(array=w435, new element=w426, index (row)=w433) -> (w434:string[][])  [unwired: 1 in]
        n211 = property on="script" class="MCListbox (strict)"("ItemNames"=w434) -> ()  [unwired: 2 in, 2 out]
      }
      frame "removeStep" {
        n212 = property on="script" class="MCListbox (strict)"() -> ("ItemNames"=w443:string[][], "Value"=w441:i32)  [unwired: 2 in, 2 out]
        n213 = Delete From Array(array=w443, index (row)=w441) -> (array with subset deleted=w442:string[][])  [unwired: 2 in, 1 out]
        n214 = property on="script" class="MCListbox (strict)"("ItemNames"=w442) -> ()  [unwired: 2 in, 2 out]
      }
      frame "onStartClicked" {
        w463 = dbl[] [] ("time")
        n215 = local write "Locked Time"(0.0 ("Locked Time")) -> ()
        n216 = local read "tab"() -> (w460:T1)
        n217 = case shown="\"Voltage Vs Wavelength\"" w460 {
          tunnel: [u32 0 u32 0 u32 2000] -> w458
          tunnel: w450 -> [w478 w481 w486]
          tunnel: [w478 w481 w485] -> w449
          frame "Voltage Vs Time", Default {
            n218 = local write "VTGraph"(cluster{dbl[], dbl[]} {[], []} ("VTGraph")) -> ()
          }
          frame "Script" {
            n219 = local write "scriptGraph"(cluster{dbl[], dbl[]} {[], []} ("scriptGraph")) -> ()
            n220 = local write "scriptSweep"(cluster{dbl[], dbl[]}[] [] ("scriptSweep")) -> ()
          }
          frame "Voltage Vs Wavelength" {
            (unwired) string[] ["SetGratingDens", "setFIlter", "setWavelength"]
            (unwired) "setWavelength"
            n221 = property on="Sweep Results" class="MCListbox (strict)"("ItemNames"=string[][] [] ("Item Names")) -> ()  [unwired: 2 in, 2 out]
            n222 = local write "sweep"(cluster{dbl[], dbl[]}[] [] ("sweep")) -> ()
            n223 = Build Array (concatenate)(w486) -> (w485:string[])
          }
        }
        n224 = Wait (ms)(milliseconds to wait=w458) -> ()  [unwired: 1 out]
        n225 = local write "Wavelen(nm)"("From") -> ()
        n226 = Less Or Equal?(x="From", y="To") -> (x <= y?=w468:bool)
        n227 = Select(t=enum16{"ASC", "DESC"}."ASC" ("sweepType"), s=w468, f=enum16{"ASC", "DESC"}."DESC" ("sweepType")) -> (s? t:f=w453:enum16{"ASC", "DESC"})
        n228 = Tick Count (ms)() -> (millisecond timer value=w459:u32)
        n229 = property on="script" class="MCListbox (strict)"() -> ("ItemNames"=w454:string[][])  [unwired: 2 in, 2 out]
        n230 = call-poly "VariableManager.vi"("Tag"="SM_VOLTAGE" ("String")) -> ("Value out"=w470:dbl)  [unwired: 6 in, 4 out]
        n231 = Bundle By Name(cluster=w474, "graphUpdate"=w459, "startTime"=w459, "lastUpdate"=w459, "run?"=TRUE, "lastVoltage"=w470, "time"=w463, "SMVolt"=w463, "MerlinVal"=w463, "Wavlnth"=w463, "From"="From", "tab"="tab", "Test Mode"="Test Mode", "script"=w454, "sweepType"=w453, "Filter Num"=1) -> (w473:T7)
        n232 = call-poly "VariableManager.vi"("Operation"=enum16{"Get Tag", "Set Tag"}."Set Tag", "Value"=0.0, "Tag"="measurinWave") -> ()  [unwired: 4 in, 5 out]
        "Time Remaining" <- "Test Time"
      }
      frame "onAbortClicked" {
        n233 = Bundle By Name(cluster=w492, "run?"=FALSE) -> (w491:T7)
      }
      frame "exportSweep" {
        n234 = call "File Dialog"("pattern (all files)"="*.csv") -> ("selected path"=w500:path, "error out"=w499:errorcluster)  [unwired: 11 in, 2 out]
        n235 = property on="Sweep Results" class="MCListbox (strict)"() -> ("ColHdrString"=w501:string[], "ItemNames"=w502:string[][])  [unwired: 2 in, 2 out]
        n236 = Build Array (concatenate)(w501, w502) -> (w497:string[][])
        n237 = case shown="No Error" w499 {
          selector: w499 -> [_ w511]
          tunnel: w500 -> [w509 _]
          tunnel: w497 -> [w508 _]
          frame No Error {
            n238 = call-poly <vilib>:"Write To Spreadsheet File.vi"("delimiter (\\t)"="," ("delimiter (\\t)"), "2D data"=w508, "file path (dialog if empty)"=w509) -> ()  [unwired: 5 in, 1 out]
          }
          frame Error {
            n239 = call <vilib>:"Clear Errors.vi"("error in (no error)"=w511) -> ()  [unwired: 5 in, 2 out]
          }
        }
      }
      frame "portA" {
        n240 = call "EventClient_RaiseEvent.vi"("error in (no error)"=w513, "Data"="!PORTIN A" ("concatenated string"), "Event"="MerlinWrite") -> ("error out"=w512:errorcluster)  [unwired: 8 in]
      }
      frame "portD" {
        n241 = call "EventClient_RaiseEvent.vi"("error in (no error)"=w521, "Data"="!PORTIN D" ("concatenated string"), "Event"="MerlinWrite") -> ("error out"=w520:errorcluster)  [unwired: 8 in]
      }
      frame "SetGrating" {
        n242 = call "EventClient_RaiseEvent.vi"("error in (no error)"=w534, "Data"="GratingNo", "Event"=w532) -> ("error out"=w533:errorcluster)  [unwired: 8 in]
        n243 = call-poly "VariableManager.vi"("Value"=FALSE, "Tag"="SetGrating" ("String")) -> ()  [unwired: 6 in, 4 out]
      }
      frame "SetGratingDens" {
        n244 = call-poly "VariableManager.vi"("Value"=FALSE, "Tag"="SetGratingDens" ("String")) -> ()  [unwired: 6 in, 4 out]
        n245 = call "EventClient_RaiseEvent.vi"("error in (no error)"=w543, "Data"="GratingDen", "Event"=w541) -> ("error out"=w542:errorcluster)  [unwired: 8 in]
      }
      frame "SetSlit" {
        n246 = call-poly "VariableManager.vi"("Operation"=enum16{"Get Tag", "Set Tag"}."Set Tag", "Tag"="currSlit") -> ()  [unwired: 6 in, 4 out]
        n247 = call-poly "VariableManager.vi"("Value"=FALSE, "Tag"="SetSlit" ("String")) -> ()  [unwired: 6 in, 4 out]
        n248 = call "EventClient_RaiseEvent.vi"("error in (no error)"=w554, "Data"="Slit", "Event"=w552) -> ("error out"=w553:errorcluster)  [unwired: 8 in]
      }
      frame "setWavelength" {
        n249 = local read "Wavelen(nm)"() -> (w562:i32)
        n250 = call-poly "VariableManager.vi"("Value"=FALSE, "Tag"="setWavelength" ("String")) -> ()  [unwired: 6 in, 4 out]
        n251 = call "EventClient_RaiseEvent.vi"("error in (no error)"=w560, "Data"=w562, "Event"=w561) -> ("error out"=w559:errorcluster)  [unwired: 8 in]
      }
      frame "setFIlter" {
        n252 = call-poly "VariableManager.vi"("Value"=FALSE, "Tag"="setFIlter" ("String")) -> ()  [unwired: 6 in, 4 out]
        n253 = call "EventClient_RaiseEvent.vi"("error in (no error)"=w570, "Data"="Filter Num", "Event"=w571) -> ("error out"=w568:errorcluster)  [unwired: 8 in]
      }
      frame "ShutterOp" {
        n254 = call-poly "VariableManager.vi"("Value"=FALSE, "Tag"="ShutterOp" ("String")) -> ()  [unwired: 6 in, 4 out]
        n255 = call "EventClient_RaiseEvent.vi"("error in (no error)"=w580, "Data"="Shutter", "Event"=w579) -> ("error out"=w577:errorcluster)  [unwired: 8 in]
      }
      frame "Reset" {
        n256 = call-poly "VariableManager.vi"("Value"=FALSE, "Tag"="Reset" ("String")) -> ()  [unwired: 6 in, 4 out]
        n257 = local read "Reset"() -> (w586:bool)
        n258 = call "EventClient_RaiseEvent.vi"("error in (no error)"=w589, "Data"=w586, "Event"=w588) -> ("error out"=w587:errorcluster)  [unwired: 8 in]
      }
      frame "setMerlin" {
        n259 = call "Stall Data Flow.vim"("value in"=w606, "milliseconds to wait"=u32 500) -> ("value out"=w594:errorcluster)  [unwired: 1 out]
        n260 = Bundle By Name(cluster=T10 {"#Stages"=enum."None", "Phase"=enum."1 Phase", "SyncMode"=enum."Int Chop Off", "Time Const"=enum.".003s", "Frequency"=0}, "#Stages"="#Filter Stages", "Phase"="Phase", "SyncMode"="SyncMode", "Time Const"="Time Const", "Frequency"="Frequency") -> (w603:T10)
        n261 = call "EventClient_RaiseEvent.vi"("error in (no error)"=w594, "Data"=w603, "Event"="setMerlin") -> ("error out"=w605:errorcluster)  [unwired: 8 in]
      }
      frame "Port set" {
        n262 = Bundle By Name(cluster=T9 {"Mono Cr"={"Port"="COM3", "baud rate"=19200, "data bits"=8, "parity"=enum."None", "stop bits"=10, "flow control"=0, "timeout"=2000}, "Merlin"={"Port"="COM4", "baud rate"=9600, "data bits"=8, "parity"=enum."None", "stop bits"=10, "flow control"=0, "timeout"=2000}} ("Settings"), "Mono Cr.Port"="Mono", "Merlin.Port"="Merlin") -> (w611:T9)
        n263 = call "LV2GSettings.vi"("Operation"=Settings_Operation."Write File", "error in (no error)"=w615, "Settings"=w611) -> ("error out"=w614:errorcluster)  [unwired: 7 in, 1 out]
      }
      frame "---------------Below are Menu Events---------------" {
        # "This State will never Execute\nIt is added just for improving code readability please do not remove this case"
      }
      frame "---------------Below are Client Events---------------" {
        # "To Handle Event Duplicate this case. If Event Does not have any data then remove\nGet Event Data and variant to data VIs"
        # "Connect Proper DataType Here"
        n264 = call "EventClient_GetEventData.vi"("error in (no error)"=w631, "reference"=w632) -> ("error out"=w630:errorcluster, "Data"=w628:variant, "reference out"=w627:T8)  [unwired: 7 in]
        n265 = Variant To Data(error in=w630, type=variant, Variant=w628) -> (error out=w629:errorcluster)  [unwired: 1 out]
      }
      frame "updateScriptSweep" {
        n266 = call "EventClient_GetEventData.vi"("error in (no error)"=w660, "reference"=w661) -> ("error out"=w659:errorcluster, "Data"=w657:variant, "reference out"=w656:T8)  [unwired: 7 in]
        n267 = Variant To Data(error in=w659, type=cluster{"wave":dbl, "smV":dbl, "mV":dbl} {"wave"=0.0, "smV"=0.0, "mV"=0.0}, Variant=w657) -> (data=w638:cluster{"wave":dbl, "smV":dbl, "mV":dbl}, error out=w658:errorcluster)
        n268 = local read "scriptSweep"() -> (w640:cluster{dbl[], dbl[]}[])
        n269 = Unbundle By Name(w638) -> ("wave"=w637:dbl, "smV"=w636:dbl, "mV"=w635:dbl)
        n270 = Index Array(array=w640, index #1=0 ("index")) -> (element #1=w642:cluster{dbl[], dbl[]}, element #2=w645:cluster{dbl[], dbl[]})  [unwired: 1 in]
        n271 = Unbundle(w642) -> (w647:dbl[], w648:dbl[])
        n272 = Unbundle(w645) -> (w646:dbl[], w649:dbl[])
        n273 = Build Array (concatenate)(w647, w637) -> (w644:dbl[])
        n274 = Build Array (concatenate)(w648, w636) -> (w652:dbl[])
        n275 = Build Array (concatenate)(w646, w637) -> (w650:dbl[])
        n276 = Build Array (concatenate)(w649, w635) -> (w651:dbl[])
        n277 = Bundle(cluster=w642, w644, w652) -> (w643:cluster{dbl[], dbl[]})
        n278 = Bundle(w650, w651) -> (w653:cluster{dbl[], dbl[]})  [unwired: 1 in]
        n279 = Build Array(w643, w653) -> (→"scriptSweep":cluster{dbl[], dbl[]}[])
      }
      frame "currGrating" {
        n280 = call "EventClient_GetEventData.vi"("error in (no error)"=w671, "reference"=w672) -> ("error out"=w670:errorcluster, "Data"=w668:variant, "reference out"=w667:T8)  [unwired: 7 in]
        n281 = Variant To Data(error in=w670, type=u32 0, Variant=w668) -> (data=w664:u32, error out=w669:errorcluster)
        n282 = local write "GratingNo"(w664) -> ()
      }
      frame "---------------Below are Subroutine states---------------" {
      }
      frame "onTimeout" {
        n283 = Unbundle By Name(w696) -> ("run?"=w695:bool, "tab"=w694:T1, "Test Mode"=w693:enum16{"Time Mode", "dV/dt Mode"}, "lastUpdate"=w692:u32)
        n284 = call-poly "VariableManager.vi"("Tag"="GratingChange?") -> ("Value out"=w687:bool)  [unwired: 7 in, 3 out]
        "gratSetup?" <- w687
        n285 = call-poly "VariableManager.vi"("Tag"="filterChange?") -> ("Value out"=w686:bool)  [unwired: 7 in, 3 out]
        "filterSetup?" <- w686
        n286 = Or(x=w687, y=w686) -> (x .or. y?=w685:bool)
        n287 = case shown="True" w695 {
          tunnel: w694 -> [_ w717]
          tunnel: w693 -> [_ _]
          tunnel: w692 -> [_ w716]
          tunnel: [w710 w713] -> w691
          tunnel: w690 -> [w710 w714]
          tunnel: w685 -> [_ w715]
          frame False {
            n288 = for {
              tunnel: string[] ["SM_VOLTAGE", "MERLIN_VALUE", "DCVoltage", "DCCurrent"] ("State Array Out") -> [w712] mode=indexing
              tunnel: [w711] -> w708 mode=indexing
              n289 = call-poly "VariableManager.vi"("Tag"=w712) -> ("Value out"=w711:dbl)  [unwired: 6 in, 4 out]
            }
            n290 = Index Array(array=w708, index #1=0 ("index")) -> (element #1=→"Source Meter Voltage":dbl, element #2=→"Merlin Voltage":dbl, element #3=→"Agilent Voltage":dbl, element #4=→"Agilent Current":dbl)  [unwired: 3 in]
          }
          frame True {
            n291 = case shown="\"Voltage Vs Wavelength\"" w717 {
              tunnel: w716 -> [_ _ _]
              tunnel: w715 -> [_ w721 w728]
              tunnel: w714 -> [w720 w723 w730]
              tunnel: [w718 w722 w729] -> w713
              frame "Voltage Vs Time", Default {
                n292 = Build Array (concatenate)(w720, "accumVTValues" ("String")) -> (w718:string[])
              }
              frame "Voltage Vs Wavelength" {
                n293 = case shown="False" w721 {
                  tunnel: w723 -> [w726 w727]
                  tunnel: [w725 w727] -> w722
                  frame False {
                    n294 = Build Array (concatenate)(w726, "updateSweepGraph" ("String")) -> (w725:string[])
                  }
                  frame True {
                  }
                }
              }
              frame "Script" {
                n295 = case shown="False" w728 {
                  tunnel: w730 -> [w731 w733]
                  tunnel: [w731 w732] -> w729
                  frame False {
                  }
                  frame True {
                    n296 = Build Array (concatenate)(w733, "executeScript" ("String")) -> (w732:string[])
                  }
                }
              }
            }
          }
        }
        n297 = for {
          tunnel: string[] ["measurinWave", "MERLIN_FEEQ", "MERLIN_VALUE"] -> [w702] mode=indexing
          tunnel: [w701] -> w683 mode=indexing
          n298 = call-poly "VariableManager.vi"("Tag"=w702) -> ("Value out"=w701:dbl)  [unwired: 6 in, 4 out]
        }
        n299 = Index Array(array=w683) -> (element #1=→"Measuring Wavelength":dbl, element #2=w681:dbl, element #3=w680:dbl)  [unwired: 3 in]
        n300 = disable-structure shown="Enabled" {
          disable-tunnel: w681 -> [w700 _]
          frame Disabled {
            n301 = local write "Frequency"(w700) -> ()
          }
          frame Enabled {
          }
        }
        n302 = local write "Merlin Voltage"(w680) -> ()
      }
      frame "accumVTValues" {
        n303 = Unbundle By Name(w742) -> ("startTime"=w748:u32, "SMVolt"=w744:dbl[], "Test Mode"=w739:enum16{"Time Mode", "dV/dt Mode"})
        n304 = Tick Count (ms)() -> (millisecond timer value=w749:u32)
        n305 = Subtract(x=w749, y=w748) -> (x-y=w750:u32)
        n306 = local read "Test Time"() -> (w747:dbl)
        n307 = Divide(x=w750, y=u32 1000) -> (x/y=w743:dbl)
        n308 = call-poly "VariableManager.vi"("Tag"="SM_VOLTAGE") -> ("Value out"=w735:dbl)  [unwired: 6 in, 4 out]
        n309 = Subtract(x=w747, y=w743) -> (x-y=w746:dbl)
        n310 = Build Array (concatenate)(w744, w735) -> (w740:dbl[])
        n311 = Bundle By Name(cluster=w742, "SMVolt"=w740) -> (w741:T7)
        n312 = case shown="\"Time Mode\", Default" w739 {
          tunnel: w746 -> [w755 _]
          frame "Time Mode", Default {
            n313 = local write "Time Remaining"(w755) -> ()
          }
          frame "dV/dt Mode" {
            n314 = local write "Time Remaining"(0.0 ("Time Remaining")) -> ()
          }
        }
        n315 = Build Array (concatenate)(w737, "updateVTGraph" ("String")) -> (w736:string[])
      }
      frame "updateVTGraph" {
        n316 = Unbundle By Name(w771) -> ("graphUpdate"=w762:u32, "startTime"=w761:u32, "SMVolt"=w770:dbl[], "lastVoltage"=w769:dbl)
        n317 = Tick Count (ms)() -> (millisecond timer value=w763:u32)
        n318 = Subtract(x=w763, y=w762) -> (x-y=w767:u32)
        n319 = Subtract(x=w763, y=w761) -> (x-y=w764:u32)
        n320 = Divide(x=w764, y=u32 1000) -> (x/y=w759:dbl)
        n321 = Greater Or Equal?(x=w767, y="Log Interval") -> (x >= y?=w760:bool)
        n322 = case shown="True" w760 {
          tunnel: w771 -> [w776 w789]
          tunnel: w770 -> [_ w788]
          tunnel: w769 -> [_ w787]
          tunnel: [w776 w784] -> w768
          tunnel: w759 -> [_ w781]
          tunnel: w758 -> [w775 w779]
          tunnel: [w775 w778] -> w757
          frame False {
          }
          frame True {
            w783 = dbl[] [] ("time")
            n323 = call "getAvarageVoltageForInterval.vi"("lastVal"=w787, "voltages"=w788) -> ("avarage"=w780:dbl)  [unwired: 9 in]
            n324 = local read "VTGraph"() -> (w785:cluster{dbl[], dbl[]})
            n325 = local write "Source Meter Voltage"(w780) -> ()
            n326 = Unbundle(w785) -> (w793:dbl[], w792:dbl[])
            n327 = Build Array (concatenate)(w779, "checkForVTAbort" ("String")) -> (w778:string[])
            n328 = Build Array (concatenate)(w793, w781) -> (w791:dbl[])
            n329 = Build Array (concatenate)(w792, w780) -> (w790:dbl[])
            n330 = Bundle(w791, w790) -> (→"VTGraph":cluster{dbl[], dbl[]})  [unwired: 1 in]
            n331 = Tick Count (ms)() -> (millisecond timer value=w782:u32)
            n332 = Bundle By Name(cluster=w789, "time"=w783, "SMVolt"=w783, "graphUpdate"=w782, "lastVoltage"=w780) -> (w784:T7)
          }
        }
      }
      frame "checkForVTAbort" {
        n333 = Unbundle By Name(w800) -> ("Test Mode"=w801:enum16{"Time Mode", "dV/dt Mode"})  [unwired: 1 out]
        n334 = case shown="\"dV/dt Mode\"" w801 {
          tunnel: w800 -> [w806 w822]
          tunnel: [w806 w822] -> w799
          tunnel: [w805 w815] -> w797
          frame "Time Mode", Default {
            n335 = local read "Time Remaining"() -> (w807:dbl)
            n336 = Greater Or Equal To 0?(x=w807) -> (x >= 0?=w805:bool)
          }
          frame "dV/dt Mode" {
            n337 = local read "VTGraph"() -> (w814:cluster{dbl[], dbl[]})
            n338 = local read "Log Interval"() -> (w808:u32)
            n339 = Unbundle(w814) -> (w812:dbl[], w813:dbl[])
            n340 = local read "Locked Time"() -> (w816:dbl)
            n341 = call "getdVbydt.vi"("times"=w812, "voltages"=w813) -> ("dV/dT"=w811:dbl)  [unwired: 7 in, 2 out]
            "dV/dt" <- w811
            n342 = Divide(x=w808, y=1000.0 ("x")) -> (x/y=w810:dbl)
            n343 = Less Or Equal?(x=w811, y="Target dV/dt") -> (x <= y?=w821:bool)
            n344 = Add(x=w810, y=w816) -> (x+y=w820:dbl)
            n345 = case shown="False" w821 {
              tunnel: [0.0 ("Locked Time") w824] -> w818
              tunnel: w820 -> [_ w824]
              frame False {
              }
              frame True {
              }
            }
            "Locked Time" <- w818
            n346 = Greater Or Equal?(x="Lock In time", y=w818) -> (x >= y?=w815:bool)
          }
        }
        n347 = Build Array (concatenate)(w796, "checkNextTest" ("String")) -> (w795:string[])
        n348 = Bundle By Name(cluster=w799, "run?"=w797) -> (w798:T7)
      }
      frame "checkNextTest" {
        n349 = Unbundle By Name(w833) -> ("run?"=w832:bool, "tab"=w826:T1)
        n350 = Build Array (concatenate)(w828, "onStartClicked" ("String")) -> (w829:string[])
        n351 = Equal?(x=w826, y="Perform Test After") -> (x = y?=w831:bool)
        n352 = case shown="False" w832 {
          tunnel: w831 -> [w839 _]
          tunnel: w828 -> [w843 w844]
          tunnel: [w842 w844] -> w830
          tunnel: w829 -> [w841 _]
          tunnel: w826 -> [w838 _]
          tunnel: "Perform Test After" -> [w840 _]
          frame False {
            n353 = Select(t=w843, s=w839, f=w841) -> (s? t:f=w842:string[])
            n354 = Select(t=w838, s=w839, f=w840) -> (s? t:f=w837:T1)
            n355 = local write "tab"(w837) -> ()
          }
          frame True {
          }
        }
      }
      frame "updateSweepGraph" {
        n356 = Unbundle By Name(w857) -> ("graphUpdate"=w860:u32)
        n357 = Tick Count (ms)() -> (millisecond timer value=w848:u32)
        n358 = Subtract(x=w848, y=w860) -> (x-y=w861:u32)
        n359 = call-poly "VariableManager.vi"("Tag"="setWavelength") -> ()  [unwired: 7 in, 4 out]
        n360 = for {
          tunnel: string[] ["SM_VOLTAGE", "MERLIN_VALUE"] ("State Array Out") -> [w866] mode=indexing
          tunnel: [w865] -> w852 mode=indexing
          n361 = call-poly "VariableManager.vi"("Tag"=w866) -> ("Value out"=w865:dbl)  [unwired: 6 in, 4 out]
        }
        n362 = Greater Or Equal?(x=w861, y="Settling Time (ms)") -> (x >= y?=w858:bool)
        n363 = And(x=w858, y=TRUE) -> (x .and. y?=w847:bool)
        n364 = Index Array(array=w852, index #1=0 ("index")) -> (element #1=w850:dbl, element #2=w849:dbl)  [unwired: 1 in]
        n365 = case shown="True" w847 {
          tunnel: w857 -> [w889 w898]
          tunnel: [w882 w897] -> w856
          tunnel: w855 -> [w890 w899]
          tunnel: [w880 w899] -> w854
          tunnel: w850 -> [_ w892]
          tunnel: w849 -> [_ w891]
          tunnel: w848 -> [w875 _]
          frame True {
            w881 = dbl[] [] ("SMVolt")
            n366 = Unbundle By Name(w889) -> ("SMVolt"=w884:dbl[], "MerlinVal"=w883:dbl[])
            n367 = local read "sweep"() -> (w888:cluster{dbl[], dbl[]}[])
            n368 = Index Array(array=w888, index=0) -> (element=w873:cluster{dbl[], dbl[]})
            n369 = local read "Wavelen(nm)"() -> (w868:i32)
            n370 = call "AvarageSamples.vi"("samples"=w884) -> ()  [unwired: 10 in, 1 out]
            n371 = call "AvarageSamples.vi"("samples"=w883) -> ("Avg"=w874:dbl)  [unwired: 10 in]
            n372 = Unbundle(w873) -> (w886:dbl[], w885:dbl[])
            n373 = Build Array (concatenate)(w886, w868) -> (w869:dbl[])
            n374 = Build Array (concatenate)(w885, w874) -> (w872:dbl[])
            n375 = Bundle By Name(cluster=w889, "SMVolt"=w881, "MerlinVal"=w881, "graphUpdate"=w875) -> (w882:T7)
            n376 = Build Array(w869, w872) -> (w878:dbl[][])
            n377 = Number To Fractional String(number=w878, width (-)=i16 7) -> (F-format string=w877:string[][])  [unwired: 2 in]
            n378 = Transpose 2D Array(2D array=w877) -> (transposed array=w876:string[][])
            n379 = Bundle(cluster=w873, w869, w872) -> (w871:cluster{dbl[], dbl[]})
            n380 = Build Array (concatenate)(w890, "updateSweep") -> (w880:string[])
            n381 = property on="Sweep Results" class="MCListbox (strict)"("ItemNames"=w876) -> ()  [unwired: 2 in, 2 out]
            n382 = Build Array(w871) -> (→"sweep":cluster{dbl[], dbl[]}[])
          }
          frame False {
            n383 = Unbundle By Name(w898) -> ("SMVolt"=w896:dbl[], "MerlinVal"=w895:dbl[])
            n384 = Build Array (concatenate)(w896, w892) -> (w894:dbl[])
            n385 = Build Array (concatenate)(w895, w891) -> (w893:dbl[])
            n386 = Bundle By Name(cluster=w898, "SMVolt"=w894, "MerlinVal"=w893) -> (w897:T7)
          }
        }
        n387 = local write "Source Meter Voltage"(w850) -> ()
        n388 = local write "Merlin Voltage"(w849) -> ()
      }
      frame "updateSweep" {
        n389 = Unbundle By Name(w920) -> ("SMVolt"=w918:dbl[], "MerlinVal"=w917:dbl[], "sweepType"=w909:enum16{"ASC", "DESC"}, "From"=w908:i32)
        n390 = local read "To"() -> (w906:i32)
        n391 = case shown="\"DESC\"" w909 {
          tunnel: w908 -> [w928 w947]
          tunnel: "Step" -> [w927 w951]
          tunnel: [w926 w950] -> w904
          tunnel: w906 -> [w932 w949]
          tunnel: [w931 w948] -> w905
          tunnel: w903 -> [w925 w945]
          tunnel: [w924 w944] -> w902
          tunnel: w901 -> [w923 w943]
          tunnel: [w923 w942] -> w900
          frame "DESC" {
            n392 = Less Or Equal?(x=w932, y=w928) -> (x <= y?=w931:bool)
            n393 = call-poly "VariableManager.vi"("Tag"="setWavelength") -> ("Value out"=w929:bool)  [unwired: 7 in, 3 out]
            n394 = case shown="True" w929 {
              tunnel: w928 -> [w934 w939]
              tunnel: w927 -> [_ w938]
              tunnel: [w934 w937] -> w926
              tunnel: w925 -> [w933 w936]
              tunnel: [w933 w935] -> w924
              frame False {
              }
              frame True {
                n395 = Subtract(x=w939, y=w938) -> (x-y=w937:dbl)
                n396 = call "setWavelenght.vi"("String"="setWavelength", "error in (no error)"=w936) -> ("error out"=w935:errorcluster)  [unwired: 9 in]
              }
            }
          }
          frame "ASC" {
            n397 = call-poly "VariableManager.vi"("Tag"="setWavelength") -> ()  [unwired: 7 in, 4 out]
            n398 = Greater Or Equal?(x=w949, y=w947) -> (x >= y?=w948:bool)
            n399 = case shown="True" TRUE {
              tunnel: w951 -> [_ w962]
              tunnel: [w954 w958] -> w950
              tunnel: w947 -> [w954 w961]
              tunnel: w945 -> [w953 w956]
              tunnel: [w953 w956] -> w944
              tunnel: w943 -> [w952 w960]
              tunnel: [w952 w959] -> w942
              frame False {
              }
              frame True {
                (unwired) string[] ["SetGratingDens", "setFIlter", "setWavelength", "setWavelength"]
                n400 = Add(x=w961, y=w962) -> (x+y=w958:dbl)
                n401 = call "FIlter Selection.vi"("Measuring Wavelength"=w958) -> ("Filter Num"=w957:i32)  [unwired: 10 in]
                n402 = local write "Filter Num"(w957) -> ()
                n403 = Build Array (concatenate)(w960, "setWavelength") -> (w959:string[])
              }
            }
          }
        }
        n404 = for {
          tunnel: string[] ["SM_VOLTAGE", "MERLIN_VALUE"] ("State Array Out") -> [w964] mode=indexing
          tunnel: [w963] -> w913 mode=indexing
          n405 = call-poly "VariableManager.vi"("Tag"=w964) -> ("Value out"=w963:dbl)  [unwired: 6 in, 4 out]
        }
        n406 = Index Array(array=w913, index #1=0 ("index")) -> (element #1=w911:dbl, element #2=w910:dbl)  [unwired: 1 in]
        n407 = Build Array (concatenate)(w918, w911) -> (w916:dbl[])
        n408 = Build Array (concatenate)(w917, w910) -> (w915:dbl[])
        n409 = local write "Measuring Wavelength"(w904) -> ()
        n410 = Bundle By Name(cluster=w920, "SMVolt"=w916, "MerlinVal"=w915, "run?"=w905, "From"=w904) -> (w919:T7)
        n411 = local write "Wavelen(nm)"(w904) -> ()
      }
      frame "executeScript" {
        n412 = Unbundle By Name(w971) -> ("script"=w967:string[][], "lastUpdate"=w979:u32)
        n413 = call "executeScript.vi"("script"=w967, "lastUpdate"=w979, "error in (no error)"=w981) -> ("scriptOut"=w966:string[][], "lastUpdate 2"=w970:u32, "error out"=w980:errorcluster)  [unwired: 5 in]
        n414 = Build Array (concatenate)(w985, "updateScriptGraph" ("String")) -> (w973:string[])
        n415 = for {
          tunnel: string[] ["DCVoltage", "DCCurrent", "SM_VOLTAGE"] ("State Array Out") -> [w1001] mode=indexing
          tunnel: [w1000] -> w977 mode=indexing
          n416 = call-poly "VariableManager.vi"("Tag"=w1001) -> ("Value out"=w1000:dbl)  [unwired: 6 in, 4 out]
        }
        n417 = Empty Array?(array=w966) -> (empty?=w968:bool)
        n418 = Not(x=w968) -> (.not. x?=w965:bool)
        n419 = Index Array(array=w977, index #1=0 ("index")) -> (element #1=w974:dbl, element #2=w975:dbl, element #3=w969:dbl)  [unwired: 2 in]
        n420 = local write "Agilent Voltage"(w974) -> ()
        n421 = local write "Agilent Current"(w975) -> ()
        n422 = local write "Source Meter Voltage"(w969) -> ()
        n423 = case shown="False" w965 {
          frame False {
            w994 = 0 ("index (row)")
            n424 = local read "scriptSweep"() -> (w986:cluster{dbl[], dbl[]}[])
            n425 = Index Array(array=w986, index #1=0 ("index")) -> (element #1=w988:cluster{dbl[], dbl[]}, element #2=w989:cluster{dbl[], dbl[]})  [unwired: 1 in]
            n426 = Unbundle(w988) -> (w991:dbl[], w993:dbl[])
            n427 = Unbundle(w989) -> (w992:dbl[])  [unwired: 1 out]
            n428 = Delete From Array(array=w991, index=w994) -> (array with subset deleted=w995:dbl[])  [unwired: 1 in, 1 out]
            n429 = Delete From Array(array=w993, index=w994) -> (array with subset deleted=w996:dbl[])  [unwired: 1 in, 1 out]
            n430 = Delete From Array(array=w992, index=w994) -> (array with subset deleted=w997:dbl[])  [unwired: 1 in, 1 out]
            n431 = Bundle(w995, w996) -> (w998:cluster{dbl[], dbl[]})  [unwired: 1 in]
            n432 = Bundle(w995, w997) -> (w999:cluster{dbl[], dbl[]})  [unwired: 1 in]
            n433 = Build Array(w998, w999) -> (w990:cluster{dbl[], dbl[]}[])
            n434 = local write "scriptSweep"(w990) -> ()
          }
          frame True {
          }
        }
        n435 = Bundle By Name(cluster=w971, "script"=w966, "lastUpdate"=w970, "run?"=w965) -> (w982:T7)
      }
      frame "updateScriptGraph" {
        n436 = Unbundle By Name(w1010) -> ("startTime"=w1014:u32, "time"=w1008:dbl[], "SMVolt"=w1007:dbl[], "graphUpdate"=w1002:u32)
        n437 = Tick Count (ms)() -> (millisecond timer value=w1003:u32)
        n438 = Subtract(x=w1003, y=w1002) -> (x-y=w1013:u32)
        n439 = Subtract(x=w1003, y=w1014) -> (x-y=w1016:u32)
        n440 = Greater Or Equal?(x=w1013, y="Script Avg Interval") -> (x >= y?=w1011:bool)
        n441 = Divide(x=w1016, y=u32 1000) -> (x/y=w1006:dbl)
        n442 = call-poly "VariableManager.vi"("Tag"="SM_VOLTAGE" ("String")) -> ("Value out"=w1004:dbl)  [unwired: 6 in, 4 out]
        n443 = case shown="False" w1011 {
          tunnel: w1008 -> [w1028 _]
          tunnel: w1007 -> [w1027 w1039]
          tunnel: w1006 -> [w1026 w1035]
          tunnel: w1004 -> [w1025 w1033]
          tunnel: w1010 -> [w1024 w1038]
          tunnel: [w1023 w1037] -> w1009
          tunnel: w1003 -> [_ w1036]
          frame False {
            n444 = Build Array (concatenate)(w1028, w1026) -> (w1022:dbl[])
            n445 = Build Array (concatenate)(w1027, w1025) -> (w1021:dbl[])
            n446 = Bundle By Name(cluster=w1024, "time"=w1022, "SMVolt"=w1021) -> (w1023:T7)
          }
          frame True {
            w1031 = dbl[] []
            # "smV/Time\nmerlinV/wavelen\nsmV/wavelen"
            n447 = local read "scriptGraph"() -> (w1030:cluster{dbl[], dbl[]})
            n448 = Build Array (concatenate)(w1039, w1033) -> (w1034:dbl[])
            n449 = Unbundle(w1030) -> (w1043:dbl[], w1040:dbl[])
            n450 = call "AvarageSamples.vi"("samples"=w1034) -> ("Avg"=w1032:dbl)  [unwired: 10 in]
            n451 = Build Array (concatenate)(w1043, w1035) -> (w1042:dbl[])
            n452 = Build Array (concatenate)(w1040, w1032) -> (w1041:dbl[])
            n453 = Bundle By Name(cluster=w1038, "graphUpdate"=w1036, "time"=w1031, "SMVolt"=w1031) -> (w1037:T7)
            n454 = Bundle(cluster=w1030, w1042, w1041) -> (→"scriptGraph":cluster{dbl[], dbl[]})
          }
        }
      }
      frame "---------------Below are Error Handling VIs---------------" {
      }
      frame "Error" {
        n455 = Call Chain() -> (call chain=w1059:string[])
        n456 = for {
          tunnel: w1059 -> [w1067] mode=indexing
          shift-right: [w1065] -> w1056
          shift-left: "" -> [w1068]
          n457 = Concatenate Strings(w1068, w1067, " -> ") -> (w1065:string)
        }
        n458 = Unbundle By Name(w1052) -> ("code"=w1054:i32, "source"=w1053:string)
        n459 = Match Pattern(string=w1053, regular expression=":") -> (before substring=w1057:string, after substring=w1061:string)  [unwired: 1 in, 2 out]
        n460 = Format Into String(format string="Error Occured In\"%s\" state of \"%s\" VI\nError Code: %d\nError Description: \"%s\"", w1057, w1056, w1054, w1061) -> (resulting string=w1060:string)  [unwired: 2 in, 1 out]
        n461 = One Button Dialog(message=w1060) -> ()  [unwired: 1 in, 1 out]
      }
    }
    n462 = Equal?(x="Exit", y=w29) -> (x = y?=w36:bool)
    "Quit" <- w36
    n463 = call "Error Handler.vi"("Current State"=w33, "error in (no error)"=w30, "Msg Queue In"=w34) -> ("error out"=w31:errorcluster, "Msg Queue Out"=w35:string[])  [unwired: 7 in]
    n464 = Wait (ms)(milliseconds to wait=u32 100) -> ()  [unwired: 1 out]
  }
  "error out" <- w16
  n465 = disable-structure shown="Disabled" {
    frame Disabled {
    }
    frame Enabled {
    }
  }
  n466 = property class="App"(error in=w16) -> ("App.Kind"=w15:T6)  [unwired: 1 in, 2 out]
  n467 = Equal?(x=w15, y=T6."Run Time System") -> (x = y?=w13:bool)
  n468 = Quit LabVIEW(quit? (T)=w13) -> ()
